vi "wfstr2file.vi"(4 "error in":errorcluster, 5 "Array":string[][](array[string]), 7 "Byte Stream File Refnum":refnum<file>) -> (0 "error out":errorcluster, 3 "Byte Stream File Refnum 2":refnum<file>)   [LabVIEW 2010]
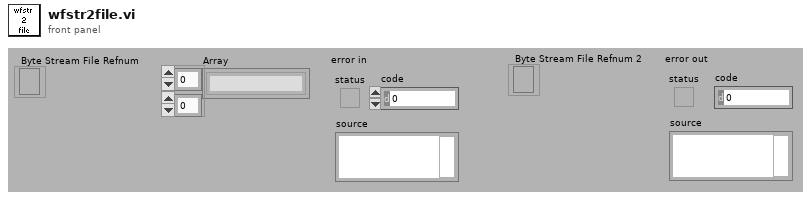
[diagram p1: front panel]
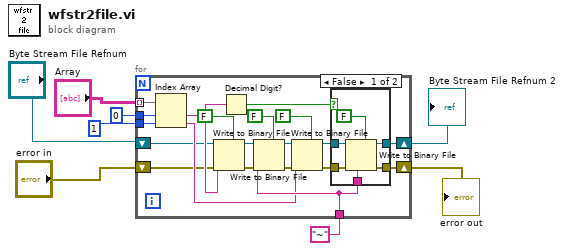
[diagram p0: block diagram]
diagram:
  n1 = for {
    tunnel: "Array" -> [w28] mode=indexing
    tunnel: 0 -> [w27]
    tunnel: 1 -> [w26]
    tunnel: "~" -> [w23]
    shift-right: [w17] -> w5
    shift-left: "Byte Stream File Refnum" -> [w21]
    shift-right: [w12] -> w6
    shift-left: "error in" -> [w16]
    n2 = Index Array(array=w28, index #1=w27, index #2=w26) -> (element #1=w24:string, element #2=w22:string)
    n3 = Write to Binary File(file (use dialog)=w21, data=w24, error in=w16, 5:FALSE ("prepend array or string size? (T)")) -> (refnum out=w20:refnum<file>, error out=w15:errorcluster)  [unwired: 2 in, 1 out]
    n4 = Decimal Digit?(1:w24) -> (0:w25:bool)
    n5 = Write to Binary File(file (use dialog)=w20, data=w23, error in=w15, 5:FALSE ("prepend array or string size? (T)")) -> (refnum out=w19:refnum<file>, error out=w14:errorcluster)  [unwired: 2 in, 1 out]
    n6 = Write to Binary File(file (use dialog)=w19, data=w22, error in=w14, 5:FALSE ("prepend array or string size? (T)")) -> (refnum out=w18:refnum<file>, error out=w13:errorcluster)  [unwired: 2 in, 1 out]
    n7 = case shown="False" w25 {
      tunnel: w23 -> [w34 _]
      tunnel: w18 -> [w33 w36]
      tunnel: [w32 w36] -> w17
      tunnel: w13 -> [w31 w35]
      tunnel: [w30 w35] -> w12
      frame False {
        n8 = Write to Binary File(file (use dialog)=w33, data=w34, error in=w31, 5:FALSE ("prepend array or string size? (T)")) -> (refnum out=w32:refnum<file>, error out=w30:errorcluster)  [unwired: 2 in, 1 out]
      }
      frame True {
      }
    }
  }
  "error out" <- w6
  "Byte Stream File Refnum 2" <- w5
